vi "Actor Core.vi"(8 "error in":errorcluster, 11 "Stage in":refnum<class "Stage.lvclass">) -> (0 "error out":errorcluster, 3 "Actor out":refnum<class "Actor.lvclass">)   [LabVIEW 2020, in "Stage.lvlib" / "Stage.lvclass"]
doc: "(<B>Filename</B>: Actor Framework.lvlib:Actor.lvclass:Actor Core.vi)\n\nReceives messages to the actor, reacts to them, and initiates any error handling that may shut the actor down.\n\nDescendant classes may override this VI to append parallel tasks for the actor to complete while it handles messages. Overrides use the Call Parent Class Method node."
uses:
  Stage.lvclass
  C:/Program Files/National Instruments/LabVIEW 2020/vi.lib/ActorFramework/Actor/Actor.lvclass
  <vilib>/ActorFramework/Actor/Actor.lvclass
  Stage Controller/Stage Controller.lvclass
  Stage.lvclass/Stage.ctl
  Device/Device/Device.lvclass
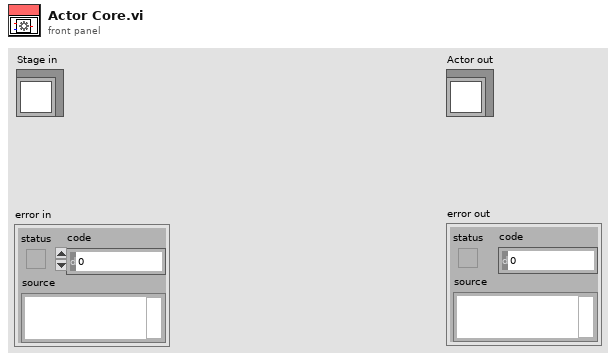
[diagram p1: front panel]
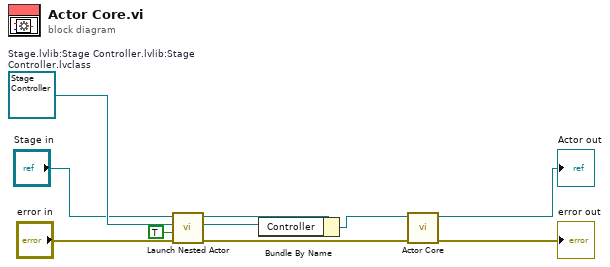
[diagram p0: block diagram]
diagram:
  w8 = refnum<class "Stage Controller.lvclass"> refnum  # Stage.lvlib:Stage Controller.lvlib:Stage Controller.lvclass
  n1 = call <vilib>:"Launch Nested Actor.vi"("error in (no error)"="error in", "Auto-stop? (T)"=TRUE, "Nested Actor"=w8, "Caller Actor in"="Stage in") -> ("error out"=w5:errorcluster, "Nested Actor's Enqueuer"=w3:refnum<class "Message Enqueuer.lvclass">, "Caller Actor out"=w4:refnum<class "Stage.lvclass">)  [unwired: 5 in]
  n2 = Bundle By Name(cluster=w4, "Controller"=w3) -> (w2:refnum<class "Stage.lvclass">)
  n3 = call-parent "Actor Core.vi"("error in"=w5, "Actor in"=w2) -> ("error out"=→"error out":errorcluster, "Actor out"=→"Actor out":refnum<class "Actor.lvclass">)  [unwired: 8 in]
